vi "oax_Separate and Scale Vibration and Tacho Channels.vi"(8 "error in (no error)":errorcluster, 9 "tacho channel index":i32, 10 "channel info in":T1[](array[typedef]) {"pregain" format="%.2f"; "weighting filter" items=["Linear", "A-weighting", "B-weighting", "C-weighting", "ITU-R 468-4", "Dolby", "CCITT", "C-message", "Wb", "Wc", "Wd", "We", "Wf", "Wh", "Wj", "Wk", "Wm", "AES17 20 kHz lowpass", "AES17 40 kHz lowpass", "AES17 20 kHz highpass", "AES17 40 kHz highpass"]; "dB reference" format="%^.1e"; "engineering units" items=["custom..."=0, "V"=1, "A"=21, "C"=30, "pC"=31, "s"=32, "-"=29, "Pa"=2, "N"=20, "g"=3, "m/s^2"=4, "m/s"=5, "m"=6, "mm/s"=12, "mm"=13, "micron/s"=14, "micron"=15, "in/s^2"=7, "in/s"=8, "in"=9, "mil/s"=10, "mil"=11, "rad/s^2"=16, "rad/s"=17, "rad"=18, "deg/s^2"=26, "deg/s"=27, "deg"=28, "RPM"=22, "cycle/s^2"=23, "Hz"=24, "cycle"=25, "strain"=19]; "sensor sensitivity" format="%#_5f"}, 11 "waveform in":waveform(dbl)[](array[waveform])) -> (0 "error out":errorcluster, 1 "tacho out":waveform(dbl), 3 "noise or vibration waveform out":waveform(dbl)[](array[waveform]))   [LabVIEW 2017]
doc: "Separates the tachometer waveform from the vibration waveform and then scales them to engineering units."
uses:
  <vilib>/addons/_NISVFA/_Shared subVIs/Controls/svc_Channel Info.ctl
  <vilib>/addons/_NISVFA/_Shared subVIs/Controls/svc_Engineering Units Text Ring.ctl
  <vilib>/addons/_NISVFA/_Shared subVIs/Controls/svc_Weighting Filter Text Ring.ctl
  <vilib>/addons/Sound and Vibration/svt_Calibration/SVL Scale Voltage to EU (N Ch - N Info).vi
  <vilib>/addons/Sound and Vibration/svt_Calibration/SVL Scale Voltage to EU (1 Ch).vi
  <vilib>/addons/_NISVFA/_Shared subVIs/Common/svc_Set SV Channel Info.vi
  <vilib>/addons/_NISVFA/_Shared subVIs/Common/svc_Set SV Channel Info (variant).vi
  <vilib>/addons/_NISVFA/_Shared subVIs/Common/SVL Set dB Reference (variant).vi
  <vilib>/addons/_NISVFA/_Shared subVIs/Common/svc_Caller VI Returned in Error Source.vi
  <vilib>/addons/_NISVFA/_Shared subVIs/Common/svc_Engineering Units to Unit Label.vi
  <vilib>/addons/_NISVFA/_Shared subVIs/Common/svc_Set dB ref if Pascal.vi
  <vilib>/addons/_NISVFA/_Shared subVIs/Common/svc_Compute Scale Factor to Convert C to EU.vi
  <vilib>/addons/_NISVFA/_Shared subVIs/Common/svc_Compute Scale Factor to Convert V to EU.vi
  <vilib>/addons/Sound and Vibration/svt_Calibration/SoundVib_Calibration.lvlib
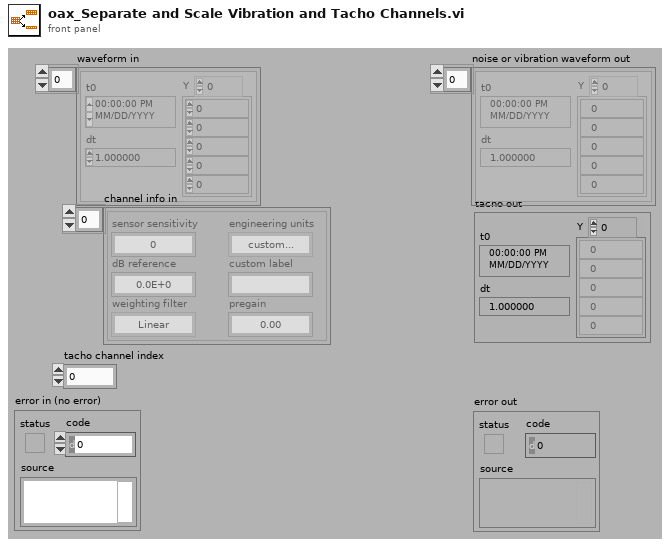
[diagram p1: front panel]
types:
  T1 = typedef "svc_Channel Info.ctl" = cluster{"sensor sensitivity":dbl, "engineering units":T2, "dB reference":dbl, "custom label":string, "weighting filter":T3, "pregain":dbl}
  T2 = typedef "svc_Engineering Units Text Ring.ctl" = u16
  T3 = typedef "svc_Weighting Filter Text Ring.ctl" = u16
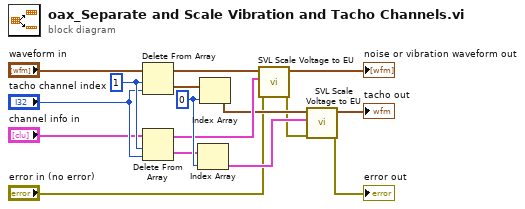
[diagram p0: block diagram]
diagram:
  w15 = 0 ("index")
  w13 = 1 ("index")
  n1 = Delete From Array(array="waveform in", length=w13, index="tacho channel index") -> (deleted portion=w10:waveform(dbl)[], array with subset deleted=w9:waveform(dbl)[])
  n2 = Delete From Array(array="channel info in", length=w13, index="tacho channel index") -> (deleted portion=w14:T1[], array with subset deleted=w7:T1[])
  n3 = Index Array(array=w14, index=w15) -> (element=w4:T1)
  n4 = Index Array(array=w10, index=w15) -> (element=w6:waveform(dbl))
  n5 = call-poly <vilib>:"SVL Scale Voltage to EU.vi"("error in (no error)"="error in (no error)", "channel info"=w7, "signals [V]"=w9) -> ("error out"=w3:errorcluster, "scaled signals [EU]"=→"noise or vibration waveform out":waveform(dbl)[])  [unwired: 6 in, 1 out]
  n6 = call-poly <vilib>:"SVL Scale Voltage to EU.vi"("error in (no error)"=w3, "channel info"=w4, "signal [V]"=w6) -> ("error out"=→"error out":errorcluster, "scaled signal [EU]"=→"tacho out":waveform(dbl))  [unwired: 6 in, 1 out]
